vi "Draw_crosshair.vi"(0 "Image IN":sgl[][](graph), 11 "White Value":sgl) -> (4 "Image OUT":sgl[][](graph))   [LabVIEW 2011]
panel:
  out "index y":i32
  out "index x":i32
  out "ny":dbl
  out "nx":dbl
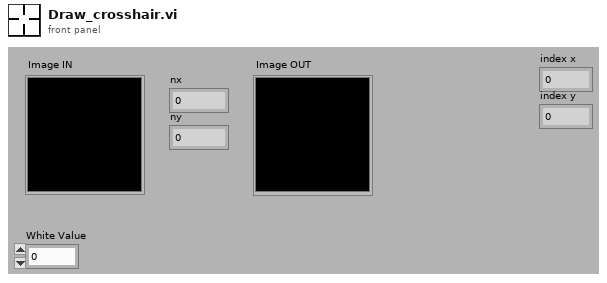
[diagram p1: front panel]
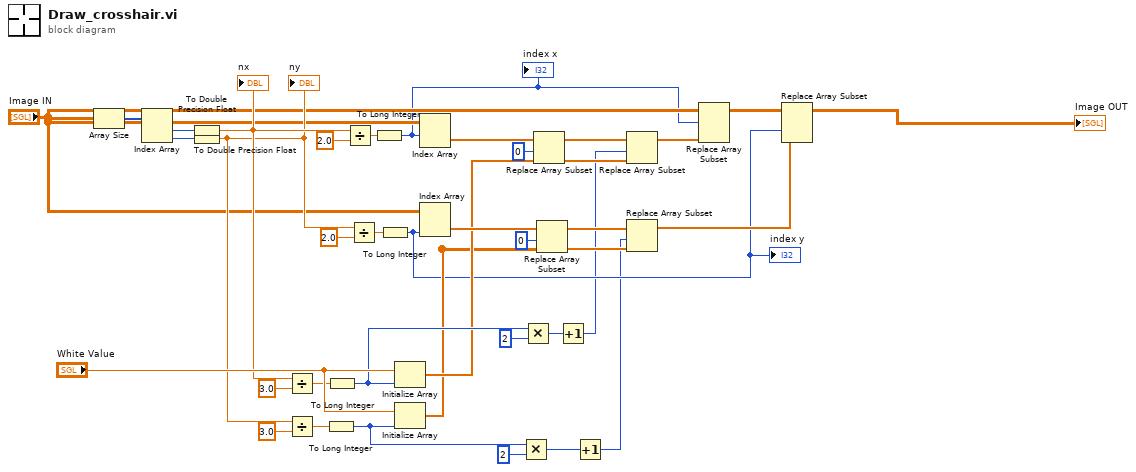
[diagram p0: block diagram]
diagram:
  n1 = Array Size(array="Image IN") -> (size(s)=w37:i32[])
  n2 = Index Array(array=w37) -> (element #1=w36:i32, element #2=w30:i32)  [unwired: 2 in]
  n3 = To Double Precision Float(number=w36) -> (double precision float=w25:dbl)
  "nx" <- w25
  n4 = To Double Precision Float(number=w30) -> (double precision float=w24:dbl)
  "ny" <- w24
  n5 = Divide(x=w25, y=3.0) -> (x/y=w28:dbl)
  n6 = Divide(x=w24, y=3.0) -> (x/y=w26:dbl)
  n7 = To Long Integer(number=w26) -> (32bit integer=w7:i32)
  n8 = To Long Integer(number=w28) -> (32bit integer=w17:i32)
  n9 = Divide(x=w25, y=2.0) -> (x/y=w33:dbl)
  n10 = Divide(x=w24, y=2.0) -> (x/y=w32:dbl)
  n11 = To Long Integer(number=w33) -> (32bit integer=w11:i32)
  "index x" <- w11
  n12 = To Long Integer(number=w32) -> (32bit integer=w3:i32)
  "index y" <- w3
  n13 = Initialize Array("White Value", w17) -> (w15:sgl[])
  n14 = Initialize Array("White Value", w7) -> (w5:sgl[])
  n15 = Index Array(array="Image IN", index (row)=w11) -> (element=w20:sgl[])  [unwired: 1 in]
  n16 = Index Array(array="Image IN", index (col)=w3) -> (element=w23:sgl[])  [unwired: 1 in]
  n17 = Multiply(x=w7, y=2) -> (x*y=w6:i32)
  n18 = Multiply(x=w17, y=2) -> (x*y=w16:i32)
  n19 = Replace Array Subset(array=w20, new element=w15, index=0) -> (w19:sgl[])
  n20 = Replace Array Subset(array=w23, new element=w5, index=0) -> (w9:sgl[])
  n21 = Increment(x=w16) -> (x+1=w1:i32)
  n22 = Increment(x=w6) -> (x+1=w2:i32)
  n23 = Replace Array Subset(array=w19, new element=w15, index=w1) -> (w10:sgl[])
  n24 = Replace Array Subset(array=w9, new element=w5, index=w2) -> (w4:sgl[])
  n25 = Replace Array Subset(array="Image IN", new element=w10, index (row)=w11) -> (w13:sgl[][])  [unwired: 1 in]
  n26 = Replace Array Subset(array=w13, new element=w4, index (col)=w3) -> (→"Image OUT":sgl[][])  [unwired: 1 in]
